vi "Validate SLSC CD Reference.vi"(8 "error in":errorcluster, 11 "ni-switch custom device in":T1 format="%.0x") -> (0 "error out":errorcluster, 3 "ni-switch custom device out":T1 format="%.0x")   [LabVIEW 2017, in "NI-SWITCH Scripting.lvlib"]
uses:
  NI-SWITCH Scripting.lvlib
  <vilib>/NI Veristand/Custom Device API/Custom Device Item Ref.ctl
  Shared/Constants.vi
  Shared/NI-SWITCH Shared.lvlib
  <vilib>/NI VeriStand/Custom Device API/Custom Device API.lvlib
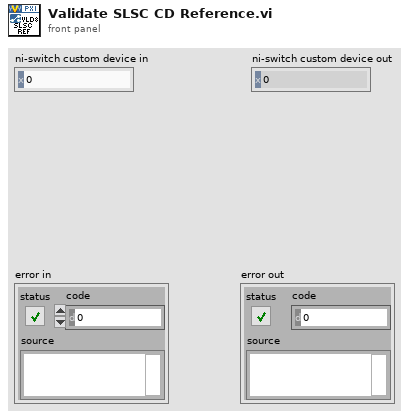
[diagram p1: front panel]
types:
  T1 = typedef "Custom Device API.lvlib/Custom Device Item Ref.ctl" = u64
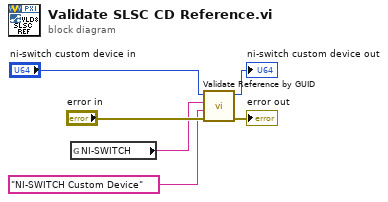
[diagram p0: block diagram]
diagram:
  n1 = global read "Constants.vi" "NI-SWITCH"() -> (w1:string)
  n2 = call "Validate Reference by GUID.vi"("error in"="error in", "name"="NI-SWITCH Custom Device" ("Name"), "guid"=w1, "slsc switch item in"="ni-switch custom device in") -> ("error out"=→"error out":errorcluster, "slsc switch item out"=→"ni-switch custom device out":T1)  [unwired: 6 in]
